vi "AnalogOutput.vi"(1 "Get/Set":bool, 2 "Analog Output (input)":T1) -> (0 "Analog Output (output)":T1)   [LabVIEW 2009]
uses:
  AnalogOutput.ctt
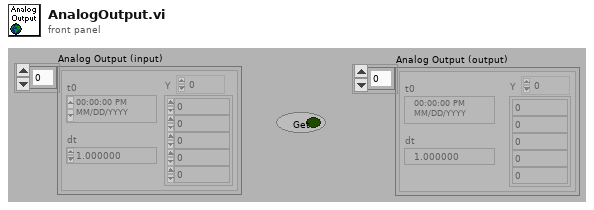
[diagram p1: front panel]
types:
  T1 = typedef "AnalogOutput.ctt" = waveform(dbl)[]
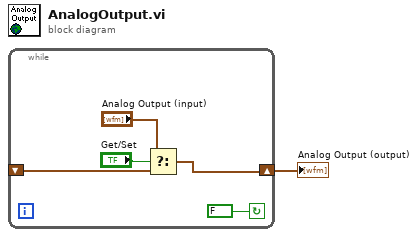
[diagram p0: block diagram]
diagram:
  n1 = while {
    shift-right: [w4] -> w1
    shift-left: _ -> [w5]
    stop <- FALSE continue-if-true
    n2 = Select(t="Analog Output (input)", s="Get/Set", f=w5) -> (s? t:f=w4:T1)
  }
  "Analog Output (output)" <- w1
